vi "Main.vi"() -> ()   [LabVIEW 2020]
uses:
  8551d84f-4896-4866-97eb-71072e9e9175.vi
panel:
  out "value out":string
  out "x-y":u32
  out "x+y":dbl
  in  "x":dbl
  in  "y":dbl
  out "First Call?: T/F":bool
  out "Array 3":i32[](array[numeric])
  out "Numeric":i32
  out "Array 2":dbl[](array[numeric])
  out "Array":i32[](array[numeric])
  in  "1D Array":i32[](array[numeric])
  out "Boolean Round":bool
  in  "Abort Button":bool
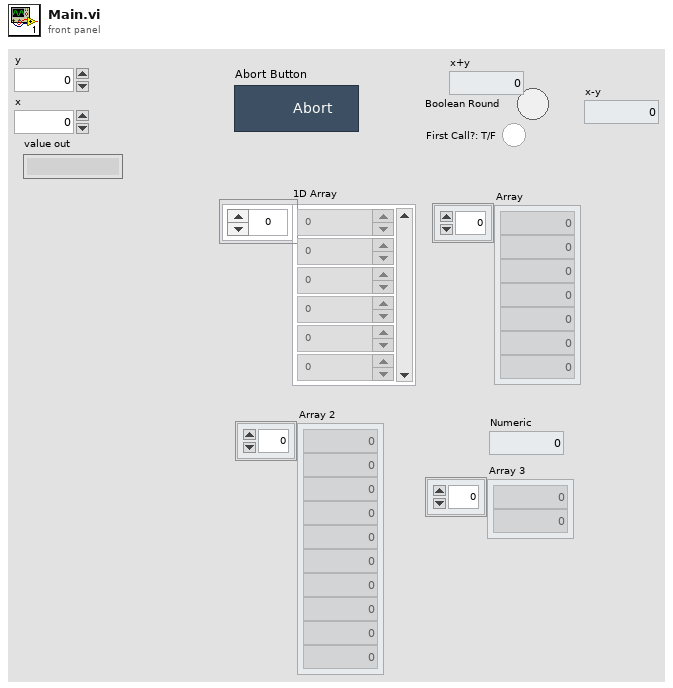
[diagram p1: front panel]
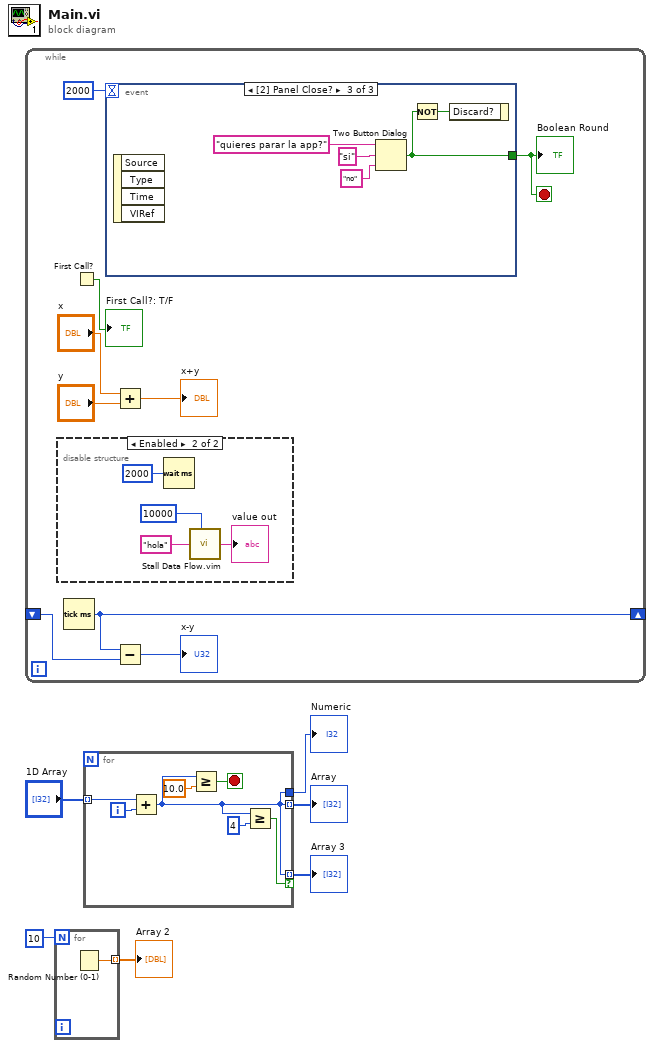
[diagram p0: block diagram]
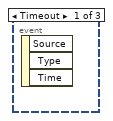
[diagram p2: hidden frame]
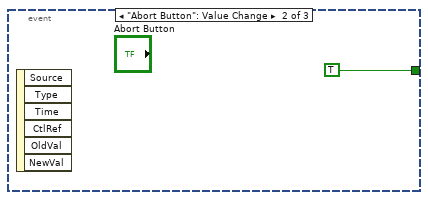
[diagram p3: hidden frame]
diagram:
  n1 = while {
    shift-right: [w10] -> _
    shift-left: _ -> [w9]
    stop <- w8 stop-if-true
    n2 = disable-structure shown="Enabled" {
      frame Disabled {
      }
      frame Enabled {
        n3 = Wait (ms)(milliseconds to wait=u32 2000) -> ()  [unwired: 1 out]
        n4 = call "Stall Data Flow.vim"("value in"="hola", "milliseconds to wait"=u32 10000) -> ("value out"=→"value out":string)  [unwired: 1 out]
      }
    }
    n5 = Tick Count (ms)() -> (millisecond timer value=w10:u32)
    n6 = First Call?() -> (First Call?: T/F=→"First Call?: T/F":bool)
    n7 = event shown="[2] Panel Close?" {
      selector: _ -> [_ _ _]
      dyn-events: _ -> [_ _ _]
      timeout: 2000 -> [_ _ _]
      tunnel: [_ TRUE ("Abort Button") w17] -> w8
      event Timeout {
        n8 = event-data() -> ()  [unwired: 1 in, 3 out]
      }
      event "Abort Button": Value Change {
        n9 = event-data() -> ()  [unwired: 1 in, 6 out]
      }
      event Panel Close? {
        n10 = event-data() -> ()  [unwired: 1 in, 4 out]
        n11 = Two Button Dialog(message="quieres parar la app?", 1:"no" ("F button name (\"Cancel\")"), 2:"si" ("T button name (\"OK\")")) -> (T button?=w17:bool)
        n12 = Not(x=w17) -> (.not. x?=w18:bool)
        n13 = event-data("Discard?"=w18) -> ()  [unwired: 1 in, 1 out]
      }
    }
    "Boolean Round" <- w8
    n14 = Add(x="x", y="y") -> (x+y=→"x+y":dbl)
    n15 = Subtract(x=w10, y=w9) -> (x-y=→"x-y":u32)
  }
  n16 = for {
    N: 10 -> [_]
    tunnel: [w26] -> w3 mode=indexing
    n17 = Random Number (0-1)() -> (number: 0 to 1=w26:dbl)
  }
  "Array 2" <- w3
  n18 = for {
    tunnel: "1D Array" -> [w32] mode=indexing
    tunnel: [w27] -> w5 mode=indexing
    tunnel: [w27] -> w2
    tunnel: [w27] -> w1 mode=indexing if=w30
    i -> [w33]
    stop <- w29 stop-if-true
    n19 = Add(x=w32, y=w33) -> (x+y=w27:i32)
    n20 = Greater Or Equal?(x=w27, y=10.0) -> (x >= y?=w29:bool)
    n21 = Greater Or Equal?(x=w27, y=4) -> (x >= y?=w30:bool)
  }
  "Array" <- w5
  "Numeric" <- w2
  "Array 3" <- w1
